vi "Export QD ShortCut.vi"() -> ()   [LabVIEW 2014]
uses:
  <resource>/dialog/lvconfig.llb/LV Config Read String.vi
  <vilib>/Utility/config.llb/Write Key (String).vi
  <vilib>/Utility/config.llb/NI_LVConfig.lvlib
panel:
  out "value":string
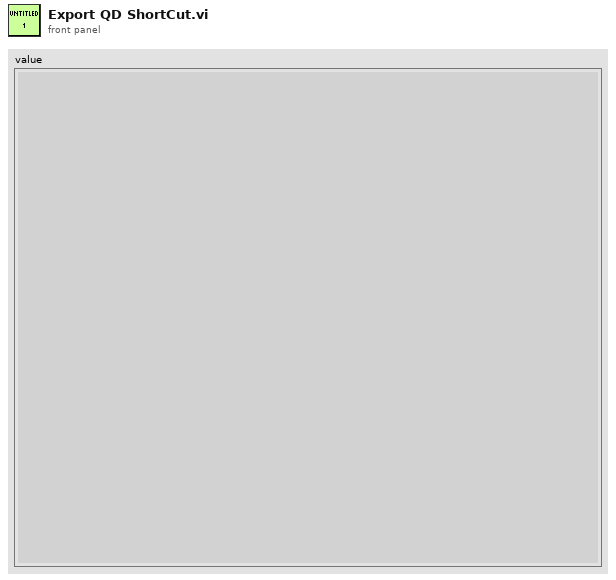
[diagram p1: front panel]
types:
  T1 = typedef "NI_LVConfig.lvlib/Config Data RefNum.ctl" = refnum<k1>
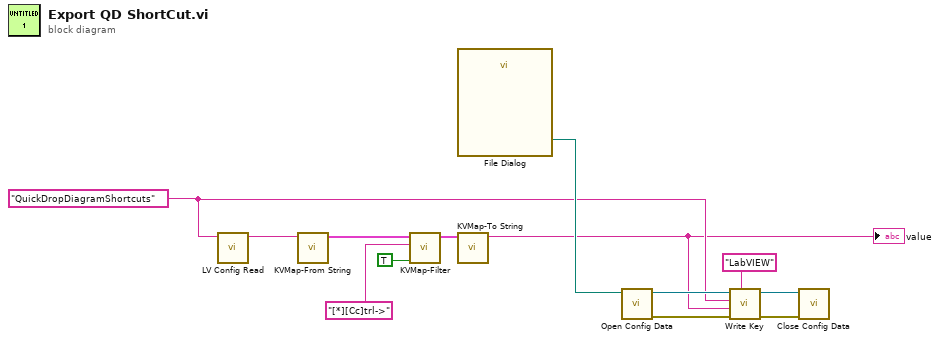
[diagram p0: block diagram]
diagram:
  w6 = "QuickDropDiagramShortcuts" ("key")
  n1 = call-poly <resource>:"LV Config Read.vi"("key"=w6) -> ("value"=w13:string)  [unwired: 4 in, 2 out]
  n2 = call "KVMap-From String.vi"("value"=w13) -> ("Cluster"=w12:cluster{string[], string[]})  [unwired: 10 in]
  n3 = call "KVMap-Filter.vi"("T->First/F->Second(F)"=TRUE, "filter"="[*][Cc]trl->", "Cluster in"=w12) -> ("Cluster out"=w11:cluster{string[], string[]})  [unwired: 8 in]
  n4 = call "File Dialog"() -> ("selected path"=w8:path)  [unwired: 12 in, 3 out]
  n5 = call "KVMap-To String.vi"("Cluster"=w11) -> ("value"=w5:string)  [unwired: 10 in]
  "value" <- w5
  n6 = call <vilib>:"Open Config Data.vi"("configuration file path"=w8) -> ("error out"=w3:errorcluster, "refnum"=w7:T1)  [unwired: 8 in, 1 out]
  n7 = call-poly <vilib>:"Write Key.vi"("section"="LabVIEW", "error in (no error)"=w3, "value"=w5, "key"=w6, "refnum"=w7) -> ("error out"=w2:errorcluster, "refnum out"=w4:T1)  [unwired: 4 in, 1 out]
  n8 = call <vilib>:"Close Config Data.vi"("error in (no error)"=w2, "refnum"=w4) -> ()  [unwired: 8 in, 2 out]
